vi "build_labels.vi"(4 "MATLAB File Directory":path, 5 "MATLAB File Prefix":string="ParseAnnularCSV_", 6 "Save MATLAB Parser?":bool, 7 "tableName":string="DataSet", 9 "Labels for saving":string[][](array[string])=[["PGAbsolutePressure", "PGpress"], ["VenturidP", "VenturidP"], ["PGVaporTemperature", "PGTvap"], ["PGLiquidTemperature", "PGTliq"], ["Window1to4dP", "W14dP"], ["Window1to7FastdP", "W17dPFast"], ["Window1to7dP", "W17dP"], ["Tinlet", "Tinlet"], ["Tsectwo", "Tsectwo"], ["TSWindow1AbsolutePressure", "TSP1"], ["TSWindow7AbsolutePressure", "TSP7"], ["DwyerdP", "DwyerdP"], ["CameraVoltage", "camera"], ["Power", "PGpower"], ["LiquidMainDiode", "mDiodeLiq"], ["LiquidControlDiode", "cDiodeLiq"], ["VaporMainDiode", "mDiodeVap"], ["VaporControlDiode", "cDiodeVap"], ["TSExteriorTemperature", "TSextTemp"], ["DSExteriorTemperature", "DSextTemp"], ["VaporMassFlow", "mdotVap"], ["VaporLineDensity", "rhoVap"], ["LiquidMassFlow", "mdotLiq"], ["LiquidLineDensity", "rhoLiq"], ["MegaTankTemperature", "MegaTankTemp"], ["MegaTankPressure", "MegaTankP"], ["SeparatorTemperature", "SepTankTemp"], ["SeparatorPressure", "SepTankP"], ["LiquidInletTemperature", "LiqInletT"], ["LiquidInletPressure", "LiqInletP"], ["UpperDevSectionTemperature", "UpDST"], ["UpperDevSectionPressure", "UpDSP"], ["LowerDevSectionPressure", "LowDSP"], ["AtmosphericPressure", "Pamb"], ["MixingTeedP", "MixTeedP"], ["PGinlet-MixingTeePressure", "PGinletTeeP"], ["PGinlet-MixingTeeTemperature", "PGinletTeeT"], ["TestSectionPressure", "TSP"], ["Tsecthree", "Tsecthree"], ["Toutlet", "Toutlet"], ["VaporInletPressure", "VapInletP"], ["VaporInletTemperature", "VapInletT"], ["WindowPowerFront", "WindowPowerFront"], ["WindowPowerBack", "WindowPowerBack"]], 11 "Analog Data Array In":T1[](array[typedef])) -> (2 "Labels":string[][](array[string]), 3 "Label Indicies":i32[](array[numeric]))   [LabVIEW 2017]
uses:
  analog_data.ctl
panel:
  out "error out":errorcluster
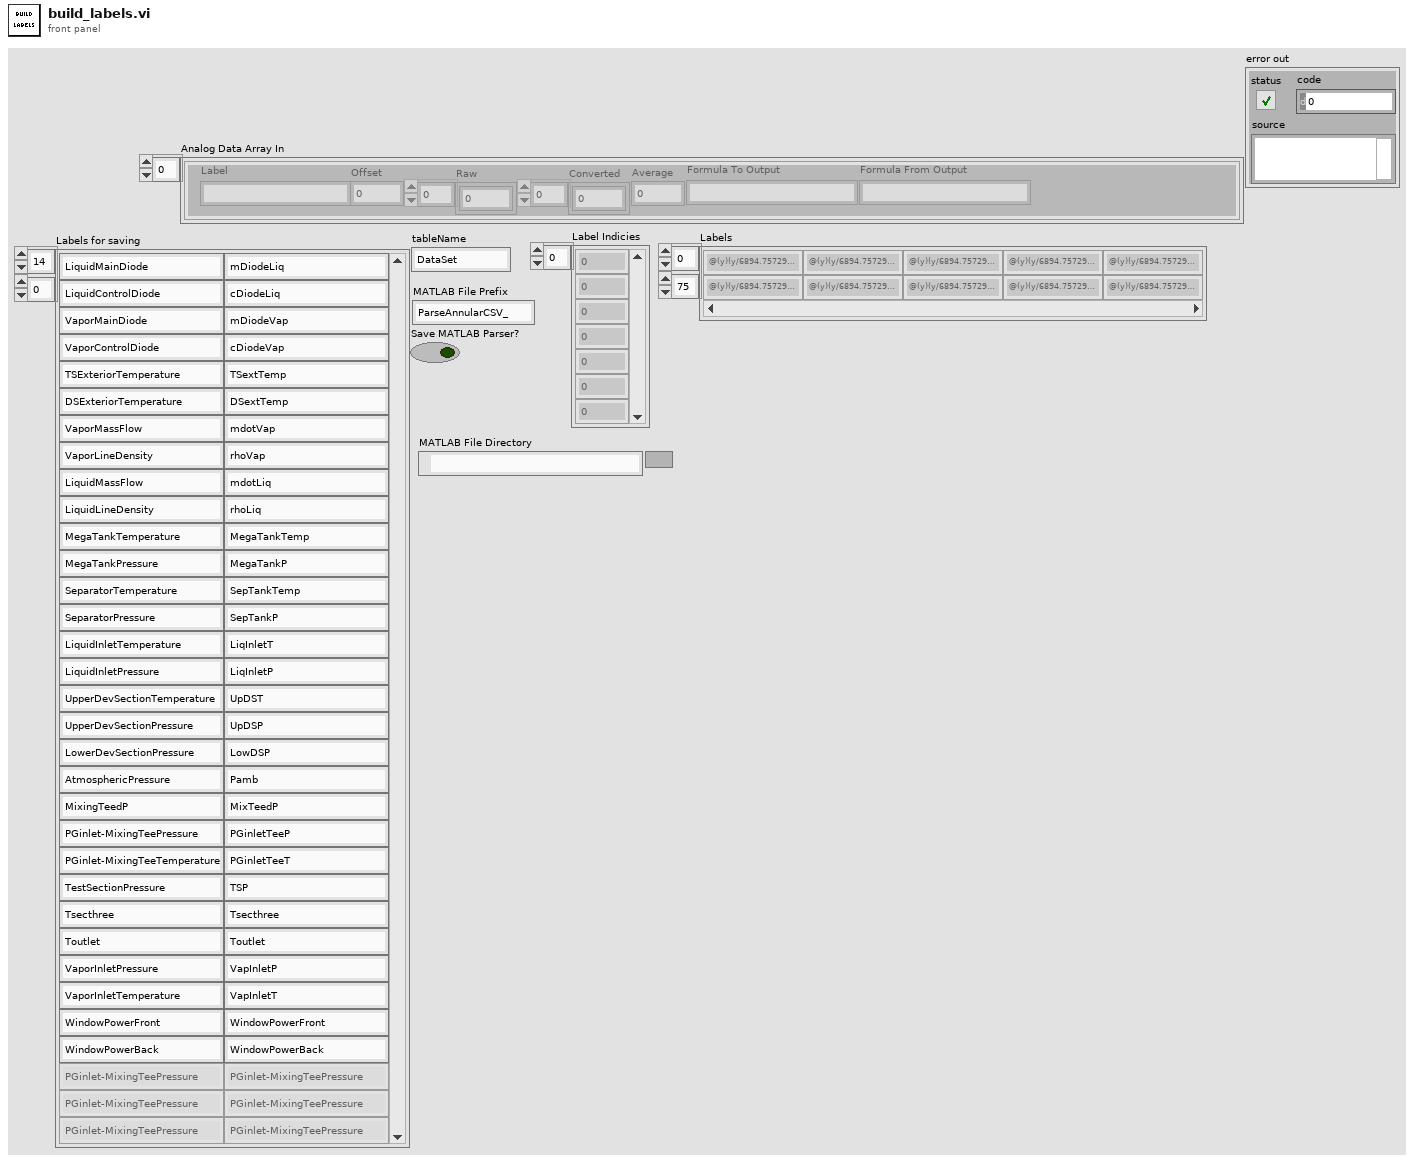
[diagram p1: front panel]
types:
  T1 = typedef "analog_data.ctl" = cluster{"Label":string, "Offset":dbl, "Raw":dbl[], "Converted":dbl[], "Average":dbl, "Formula To Output":string, "Formula From Output":string}
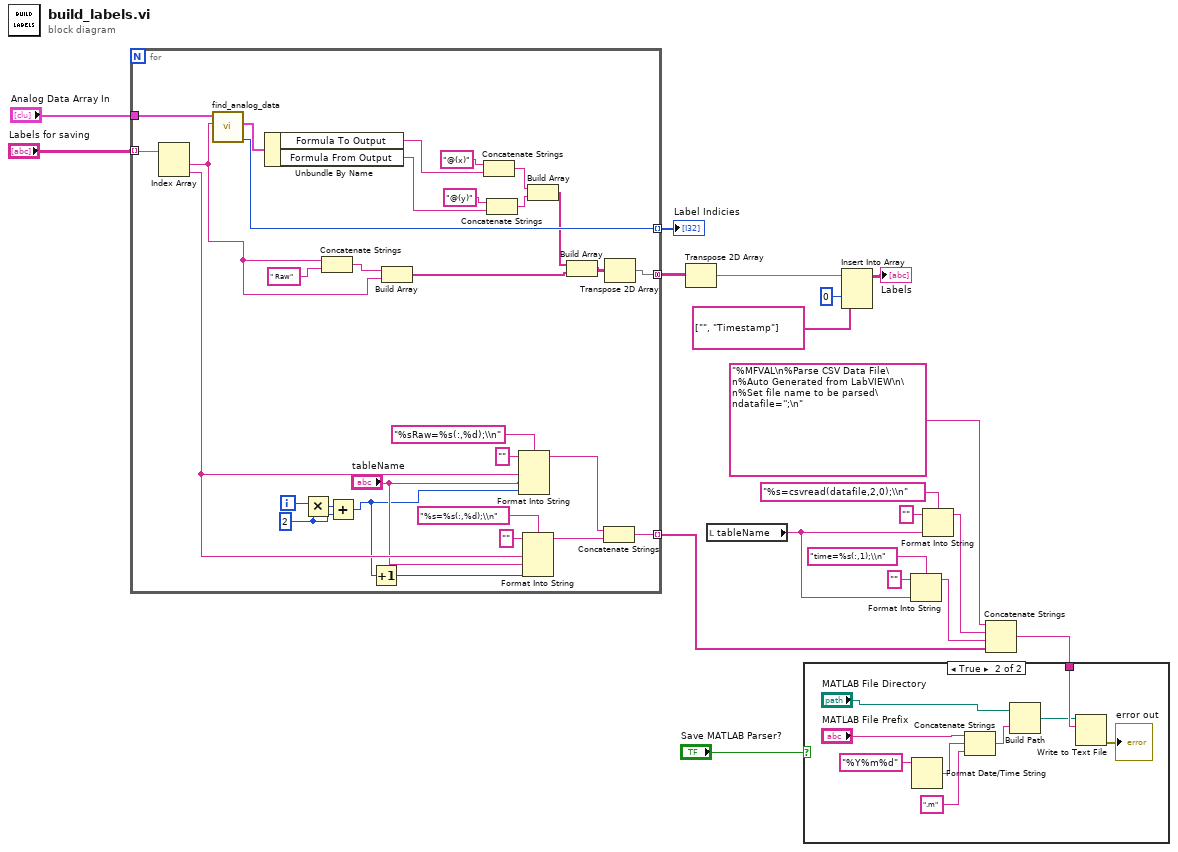
[diagram p0: block diagram]
diagram:
  n1 = for {
    tunnel: "Labels for saving" -> [w35] mode=indexing
    tunnel: [w49] -> w18 mode=indexing
    tunnel: [w43] -> w17 mode=concatenating
    tunnel: "Analog Data Array In" -> [w36]
    tunnel: [w24] -> w6 mode=indexing
    i -> [w23]
    w21 = 2 ("y")
    n2 = Index Array(array=w35) -> (element #1=w34:string, element #2=w29:string)  [unwired: 2 in]
    n3 = call "find_analog_data.vi"("Needle"=w34, "Haystack"=w36) -> ("Index"=w49:i32, "Needle Out"=w50:T1)  [unwired: 7 in, 1 out]
    n4 = Unbundle By Name(w50) -> ("Formula To Output"=w38:string, "Formula From Output"=w40:string)
    n5 = Multiply(x=w23, y=w21) -> (x*y=w22:i32)
    n6 = Concatenate Strings(w34, " Raw" ("string")) -> (w47:string)
    n7 = Add(x=w22, y=w21) -> (x+y=w20:i32)
    n8 = Increment(x=w20) -> (x+1=w27:i32)
    n9 = Build Array(w47, w34) -> (w46:string[])
    n10 = Concatenate Strings("@(x)" ("string"), w38) -> (w37:string)
    n11 = Concatenate Strings("@(y)" ("string"), w40) -> (w39:string)
    n12 = Format Into String(format string="%sRaw=%s(:,%d);\\n", initial string="", w29, "tableName", w20) -> (resulting string=w26:string)  [unwired: 1 in, 1 out]
    n13 = Format Into String(format string="%s=%s(:,%d);\\n", initial string="", w29, "tableName", w27) -> (resulting string=w25:string)  [unwired: 1 in, 1 out]
    n14 = Build Array(w37, w39) -> (w45:string[])
    n15 = Build Array(w45, w46) -> (w44:string[][])
    n16 = Concatenate Strings(w26, w25) -> (w24:string)
    n17 = Transpose 2D Array(2D array=w44) -> (transposed array=w43:string[][])
  }
  "Label Indicies" <- w18
  n18 = Transpose 2D Array(2D array=w17) -> (transposed array=w16:string[][])
  n19 = local read "tableName"() -> (w3:string)
  n20 = Insert Into Array(array=w16, index (col)=0 ("disabled index (col)"), new element=string[] ["", "Timestamp"] ("new element/subarray")) -> (→"Labels":string[][])  [unwired: 1 in]
  n21 = Format Into String(format string="time=%s(:,1);\\n", initial string="", w3) -> (resulting string=w5:string)  [unwired: 1 in, 1 out]
  n22 = Format Into String(format string="%s=csvread(datafile,2,0);\\n" ("initial string"), initial string="", w3) -> (resulting string=w9:string)  [unwired: 1 in, 1 out]
  n23 = Concatenate Strings("%MFVAL\n%Parse CSV Data File\n%Auto Generated from LabVIEW\n\n%Set file name to be parsed\ndatafile='';\n" ("initial string"), w9, w5, w6) -> (w8:string)
  n24 = case shown="True" "Save MATLAB Parser?" {
    tunnel: w8 -> [_ w59]
    frame False {
    }
    frame True {
      n25 = Format Date/Time String(time format string (%c)="%Y%m%d") -> (date/time string=w54:string)  [unwired: 2 in]
      n26 = Concatenate Strings("MATLAB File Prefix", w54, ".m" ("name or relative path")) -> (w56:string)
      n27 = Build Path(base path="MATLAB File Directory", name or relative path=w56) -> (appended path=w58:path)
      n28 = Write to Text File(file (use dialog)=w58, text=w59) -> (error out=→"error out":errorcluster)  [unwired: 2 in, 2 out]
    }
  }
